vi "fabanpassung einzug 2.vi"(2 "Device ID Out":T1(ring)) -> ()   [LabVIEW 2010]
panel:
  out "Numerisches Element":i32
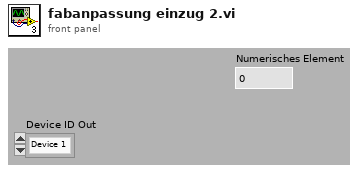
[diagram p1: front panel]
types:
  T1 = enum16{"Device 1", "Device 2", "Device 3", "Device 4", "Device 5", "Device 6", "Device 7", "Device 8"}
  T2 = enum8{"Input 1 (I1)", "Input 2 (I2)", "Input 3 (I3)", "Input 4 (I4)", "Input 5 (I5)", "Input 6 (I6)", "Input 7 (I7)", "Input 8 (I8)"}
  T3 = enum8{"Robo Interface", "Extension 1", "Extension 2", "Extension 3"}
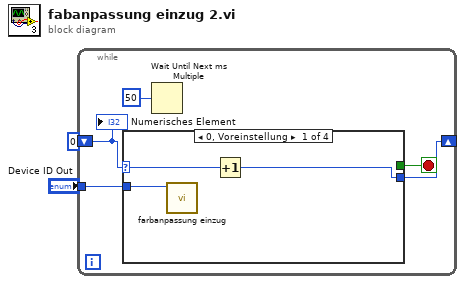
[diagram p0: block diagram]
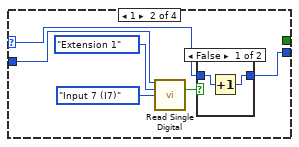
[diagram p2: hidden frame]
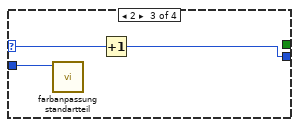
[diagram p4: hidden frame]
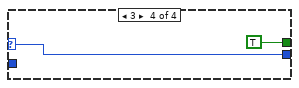
[diagram p5: hidden frame]
diagram:
  n1 = while {
    tunnel: "Device ID Out" -> [w7]
    shift-right: [w6] -> _
    shift-left: 0 -> [w3]
    stop <- w5 stop-if-true
    n2 = case shown="0, Voreinstellung" w3 {
      selector: w3 -> [w8 w11 w21 w24]
      tunnel: w7 -> [w10 w16 w22 _]
      tunnel: [w9 w12 w20 w24] -> w6
      tunnel: [_ _ _ TRUE] -> w5
      frame 0, Default {
        n3 = call "farbanpassung einzug.vi"("Device ID"=w10) -> ()  [unwired: 1 in, 10 out]
        n4 = Increment(x=w8) -> (x+1=w9:i32)
      }
      frame 1 {
        n5 = call "Read Single Digital.vi"("Device ID"=w16, "Module"=T3."Extension 1", "Digital_Input"=T2."Input 7 (I7)") -> ("Value"=w13:bool)  [unwired: 1 in, 11 out]
        n6 = case shown="FALSE" w13 {
          tunnel: [w18 w19] -> w12
          tunnel: w11 -> [w17 w19]
          frame False {
            n7 = Increment(x=w17) -> (x+1=w18:i32)
          }
          frame True {
          }
        }
      }
      frame 2 {
        n8 = call "farbanpassung standartteil.vi"("Device ID"=w22) -> ()  [unwired: 1 in, 9 out]
        n9 = Increment(x=w21) -> (x+1=w20:i32)
      }
      frame 3 {
      }
    }
    n10 = Wait Until Next ms Multiple(millisecond multiple=50) -> ()  [unwired: 1 out]
    "Numerisches Element" <- w3
  }
